vi "PCO_SetCompressionMode.vi"(8 "error in (no error)":errorcluster {"code" format="%x"}, 10 "wCompressionMode":u16, 11 "ph":u64) -> (0 "error out":errorcluster {"code" format="%x"}, 2 "ErrorMessage":i32 format="%x", 3 "ph out":u64)   [LabVIEW 2019, in "SDK.lvlib" / "StorageControl.lvlib"]
doc: "<b>Description:</b>\nSets the ram compression mode of the camera. Please check camera descriptor 3 for availability.\n\n<b>Supported camera type:</b>\npco.dimax, pco.1200, pco.1600, pco.2000, pco.4000\n\n<b>Descriptor dependency:</b>\ndwGeneralCapsDESC3"
uses:
  StorageControl.lvlib
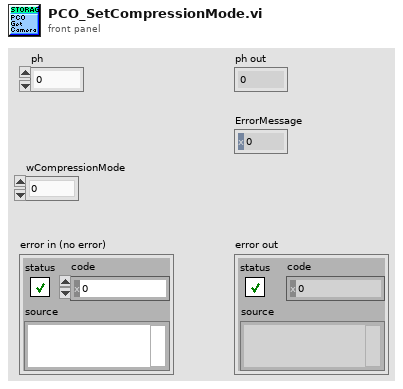
[diagram p1: front panel]
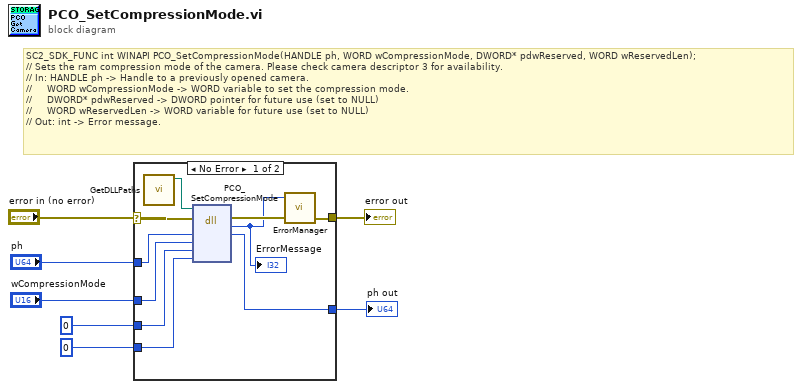
[diagram p0: block diagram]
diagram:
  # "SC2_SDK_FUNC int WINAPI PCO_SetCompressionMode(HANDLE ph, WORD wCompressionMode, DWORD* pdwReserved, WORD wReservedLen);\n// Sets the ram compression mode of the camera. Please check camera descriptor 3 for availability.\n// In: HANDLE ph -> Handle to a previously opened camera.\n//     WORD wCompressionMode -> WORD variable to set the compression mode.\n//     DWORD* pdwReserved -> DWORD pointer for future use (set to NULL)\n//     WORD wReservedLen -> WORD variable for future use (set to NULL)\n// Out: int -> Error message."
  n1 = case shown="No Error" "error in (no error)" {
    selector: "error in (no error)" -> [w15 w19]
    tunnel: "ph" -> [w17 w18]
    tunnel: [w16 w18] -> w6
    tunnel: [w13 w19] -> w5
    tunnel: "wCompressionMode" -> [w10 _]
    tunnel: u32 0 -> [w9 _]
    tunnel: u16 0 -> [w8 _]
    frame No Error {
      n2 = call "GetDLLPaths.vi"() -> ("SC2_Cam_Path"=w11:path)  [unwired: 9 in, 2 out]
      n3 = dll-call lib="?" fn="PCO_SetCompressionMode"(path in=w11, error in=w15, "ph"=w17, "wCompressionMode"=w10, "pdwReserved"=w9, "wReservedLen"=w8) -> (error out=w14:errorcluster, "return type"=w12:i32, "ph"=w16:u64)  [unwired: 4 in, 1 out]
      "ErrorMessage" <- w12
      n4 = call "ErrorManager.vi"("error in (no error)"=w14, "error code"=w12) -> ("error out"=w13:errorcluster)  [unwired: 3 in]
    }
    frame Error {
    }
  }
  "ph out" <- w6
  "error out" <- w5
